vi "Software_Version.vi"() -> ()   [LabVIEW 2013]
panel:
  in  "Software version":string
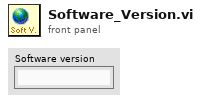
[diagram p1: front panel]
diagram:
